vi "Remove State (from Dictionaries).vi"(8 "error in (no error)":errorcluster, 10 "State":string, 11 "Channel Ref in":T1 format="%.0x") -> (0 "error out":errorcluster, 3 "Channel Ref out":T1=18446744073709551615 format="%.0x")   [LabVIEW 2017, in "Switch Scripting.lvlib"]
uses:
  Switch Scripting.lvlib
  <vilib>/NI Veristand/Custom Device API/Custom Device Item Ref.ctl
  NationalInstruments.VeriStand.SystemDefinitionAPI
  Constants.vi
  <vilib>/NI VeriStand/Custom Device API/Custom Device API.lvlib
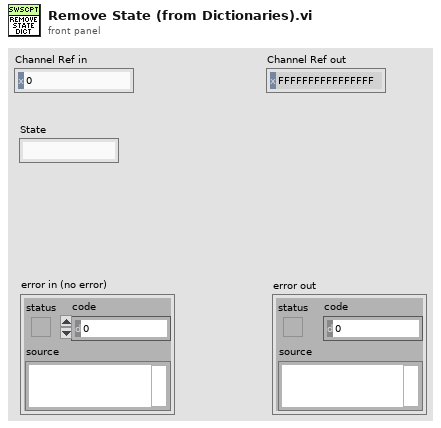
[diagram p1: front panel]
types:
  T1 = typedef "Custom Device API.lvlib/Custom Device Item Ref.ctl" = u64
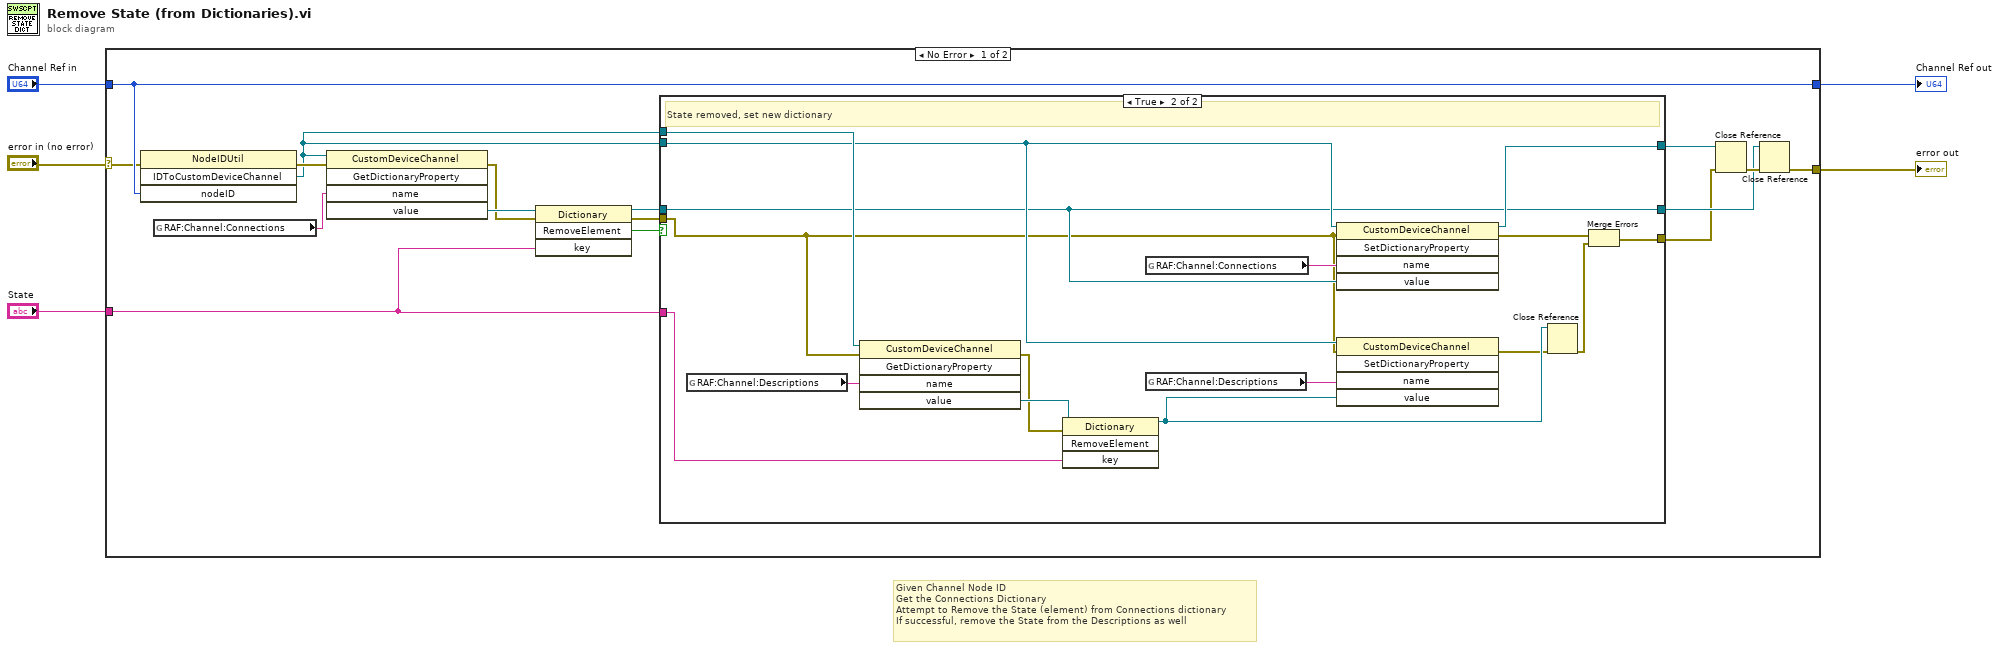
[diagram p0: block diagram]
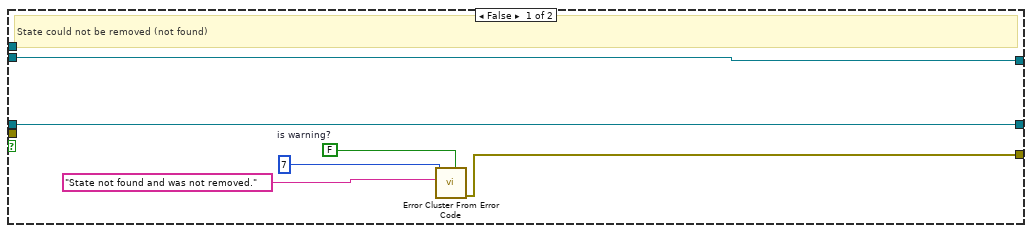
[diagram p2: hidden frame]
diagram:
  # "Given Channel Node ID\nGet the Connections Dictionary\nAttempt to Remove the State (element) from Connections dictionary\nIf successful, remove the State from the Descriptions as well"
  n1 = case shown="No Error" "error in (no error)" {
    selector: "error in (no error)" -> [w18 w45]
    tunnel: [w6 w45] -> w4
    tunnel: "Channel Ref in" -> [w19 w44]
    tunnel: [w19 w44] -> w2
    tunnel: "State" -> [w8 _]
    frame No Error {
      n2 = invoke class="NodeIDUtil" method="IDToCustomDeviceChannel"(error in=w18, "nodeID"=w19) -> (error out=w20:errorcluster, "IDToCustomDeviceChannel"=w7:refnum<k24>)  [unwired: 2 in, 2 out]
      n3 = global read "Constants.vi" "RAF:Channel:Connections"() -> (w9:string)
      n4 = invoke class="CustomDeviceChannel" method="GetDictionaryProperty"(reference=w7, error in=w20, "name"=w9) -> (error out=w16:errorcluster, "value"=w17:refnum<k24>)  [unwired: 2 in, 3 out]
      n5 = invoke class="Dictionary" method="RemoveElement"(reference=w17, error in=w16, "key"=w8) -> (reference out=w13:refnum<k24>, error out=w14:errorcluster, "RemoveElement"=w15:bool)  [unwired: 1 in, 1 out]
      n6 = case shown="True" w15 {
        tunnel: w14 -> [_ w31]
        tunnel: [w25 w33] -> w11
        tunnel: w13 -> [w24 w32]
        tunnel: [w24 w32] -> w12
        tunnel: w7 -> [w23 w35]
        tunnel: [w23 w43] -> w10
        tunnel: w8 -> [_ w37]
        tunnel: w7 -> [_ w38]
        frame False {
          w26 = FALSE  # is warning?
          # "State could not be removed (not found)"
          n7 = call <vilib>:"Error Cluster From Error Code.vi"("is warning? (False)"=w26, "error message (\"\")"="State not found and was not removed." ("error message (\"\")"), "error code (0)"=7) -> ("error out"=w25:errorcluster)  [unwired: 6 in]
        }
        frame True {
          # "State removed, set new dictionary"
          n8 = global read "Constants.vi" "RAF:Channel:Descriptions"() -> (w41:string)
          n9 = invoke class="CustomDeviceChannel" method="GetDictionaryProperty"(reference=w38, error in=w31, "name"=w41) -> (error out=w39:errorcluster, "value"=w40:refnum<k24>)  [unwired: 2 in, 3 out]
          n10 = invoke class="Dictionary" method="RemoveElement"(reference=w40, error in=w39, "key"=w37) -> (reference out=w30:refnum<k24>)  [unwired: 1 in, 3 out]
          n11 = global read "Constants.vi" "RAF:Channel:Connections"() -> (w42:string)
          n12 = global read "Constants.vi" "RAF:Channel:Descriptions"() -> (w36:string)
          n13 = invoke class="CustomDeviceChannel" method="SetDictionaryProperty"(reference=w35, error in=w31, "name"=w42, "value"=w32) -> (reference out=w43:refnum<k24>, error out=w34:errorcluster)  [unwired: 1 in, 3 out]
          n14 = invoke class="CustomDeviceChannel" method="SetDictionaryProperty"(reference=w35, error in=w31, "name"=w36, "value"=w30) -> (error out=w29:errorcluster)  [unwired: 1 in, 4 out]
          n15 = Close Reference(reference=w30, error in (no error)=w29) -> (error out=w28:errorcluster)
          n16 = Merge Errors(w34, w28) -> (w33:errorcluster)
        }
      }
      n17 = Close Reference(reference=w10, error in (no error)=w11) -> (error out=w21:errorcluster)
      n18 = Close Reference(reference=w12, error in (no error)=w21) -> (error out=w6:errorcluster)
    }
    frame Error {
    }
  }
  "Channel Ref out" <- w2
  "error out" <- w4
